vi "show QR Code.vi"() -> ()   [LabVIEW 2016, in "opSignIn.lvlib"]
uses:
  opSignIn.lvlib
panel:
  out "数值":i32
  in  "设置按钮":bool
  in  "刷新按钮":bool
  in  "单选按钮":enum32{"SignIn", "SignOut"}(radio)
  out "new picture":picture caption="新图片"
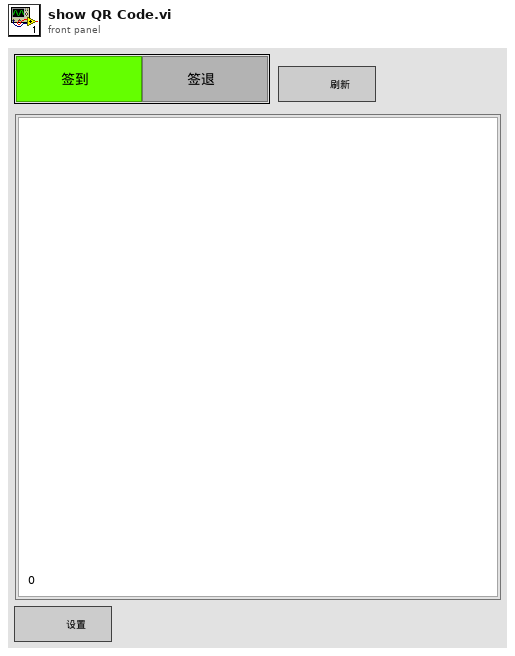
[diagram p1: front panel]
types:
  T1 = cluster{"url":string, "AccessToken":string, "mn":string, "isSignIn":bool}
  T2 = cluster{"url":string, "loginTokenRequest":cluster{"clientId":string, "clientSecret":string, "grantType":string, "password":string, "scope":string, "userName":string, "userType":string}}
  T3 = cluster{"code":string, "message":string, "timestamp":u64, "data":cluster{"bearerType":string, "oauth2Type":string, "accessToken":string, "tokenType":string, "expiresIn":u64, "refreshToken":string, "scope":string[], "tokenDetail":cluster{"dataSource":string, "username":string, "userId":string, "userType":string, "enabled":bool, "accountNonExpired":bool, "credentialsNonExpired":bool, "accountNonLocked":bool}}, "success":bool}
  T4 = cluster{"code":string, "message":string, "timestamp":u64, "success":bool, "data":cluster{"qrCodeType":string, "uuid":string, "signIn":bool, "stationMn":string, "expiration":u64, "signature":string}}
  T5 = cluster{"qrCodeType":string, "uuid":string, "signIn":bool, "stationMn":string, "expiration":u64, "signature":string}
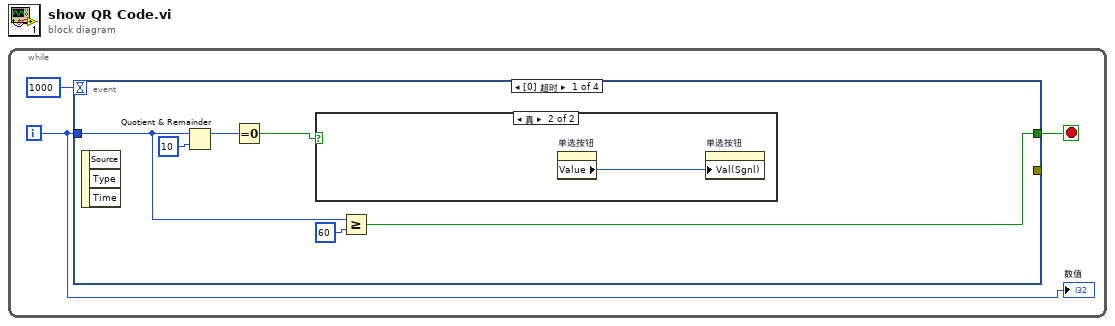
[diagram p0: block diagram]
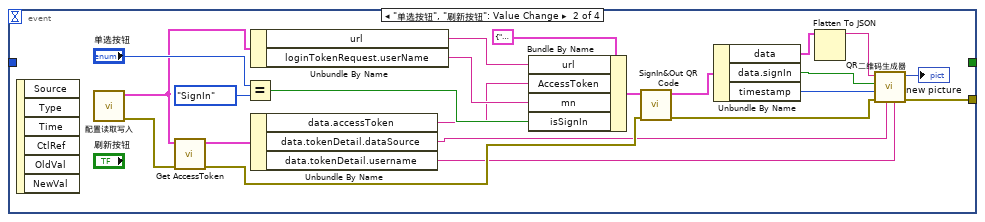
[diagram p3: hidden frame]
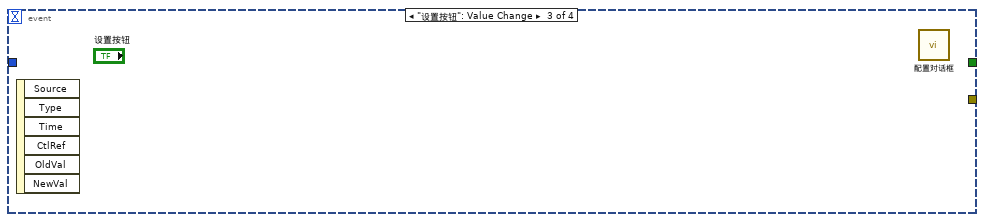
[diagram p4: hidden frame]
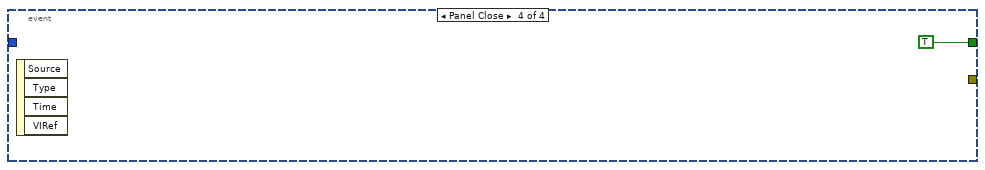
[diagram p5: hidden frame]
diagram:
  n1 = while {
    i -> [w1]
    stop <- w3 stop-if-true
    n2 = event shown="[0] 超时" {
      selector: _ -> [_ _ _ _]
      dyn-events: _ -> [_ _ _ _]
      timeout: 1000 -> [_ _ _ _]
      tunnel: [w8 _ _ TRUE] -> w3
      tunnel: [_ w16 _ _] -> _
      tunnel: w1 -> [w7 _ _ _]
      event Timeout {
        n3 = event-data() -> ()  [unwired: 1 in, 3 out]
        n4 = Quotient & Remainder(x=w7, y=10) -> (x-y*floor(x/y)=w5:i32)  [unwired: 1 out]
        n5 = Equal To 0?(x=w5) -> (x = 0?=w4:bool)
        n6 = case shown="真" w4 {
          frame False {
          }
          frame True {
            n7 = property on="单选按钮" class="RadioBtnsControl (严格)"() -> ("Value"=w10:enum32{"SignIn", "SignOut"})  [unwired: 2 in, 2 out]
            n8 = property on="单选按钮" class="RadioBtnsControl (严格)"("Val(Sgnl)"=w10) -> ()  [unwired: 2 in, 2 out]
          }
        }
        n9 = Greater Or Equal?(x=w7, y=60) -> (x >= y?=w8:bool)
      }
      event "单选按钮", "刷新按钮": Value Change {
        n10 = event-data() -> ()  [unwired: 1 in, 6 out]
        n11 = call "配置读取写入.vi"() -> ("error out"=w21:errorcluster, "配置输出"=w23:T2)  [unwired: 10 in]
        n12 = call "Get AccessToken.vi"("error in (no error)"=w21, "配置"=w23) -> ("error out"=w24:errorcluster, "response"=w25:T3)  [unwired: 8 in]
        n13 = Equal?(x="单选按钮", y=enum32{"SignIn", "SignOut"}."SignIn") -> (x = y?=w32:bool)
        n14 = Unbundle By Name(w23) -> ("url"=w13:string, "loginTokenRequest.userName"=w27:string)
        n15 = Unbundle By Name(w25) -> ("data.accessToken"=w26:string, "data.tokenDetail.dataSource"=w12:string, "data.tokenDetail.username"=w11:string)
        n16 = Bundle By Name(cluster=T1 {"url"="http://data.watersystem.com.cn:50040", "AccessToken"="equip&GbbVkGRBUSaIfhTSjiolTAP8QMM", "mn"="admin", "isSignIn"=FALSE} ("Para"), "url"=w13, "AccessToken"=w26, "mn"=w27, "isSignIn"=w32) -> (w14:T1)
        n17 = call "SignIn&Out QR Code.vi"("error in (no error)"=w24, "Para"=w14) -> ("error out"=w19:errorcluster, "response"=w28:T4)  [unwired: 8 in]
        n18 = Unbundle By Name(w28) -> ("data"=w29:T5, "data.signIn"=w18:bool, "timestamp"=w17:u64)
        n19 = Flatten To JSON(anything=w29) -> (JSON string=w20:string)  [unwired: 2 in, 1 out]
        n20 = call "QR二维码生成器.vi"("MN"=w11, "dataSource"=w12, "error in (no error)"=w19, "timestamp"=w17, "signIn"=w18, "输入文本"=w20) -> ("error out"=w16:errorcluster, "new picture"=→"new picture":picture)  [unwired: 4 in]
      }
      event "设置按钮": Value Change {
        n21 = event-data() -> ()  [unwired: 1 in, 6 out]
        n22 = call "配置对话框.vi"() -> ()  [unwired: 12 in]
      }
      event Panel Close {
        n23 = event-data() -> ()  [unwired: 1 in, 4 out]
      }
    }
    "数值" <- w1
  }
